vi "Set Scan Engine Active.vi"(8 "error in (no error)":errorcluster) -> (0 "error out":errorcluster)   [LabVIEW 2016]
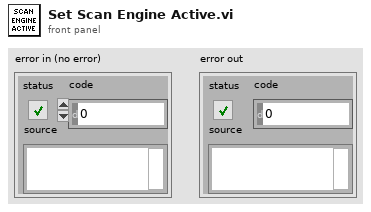
[diagram p1: front panel]
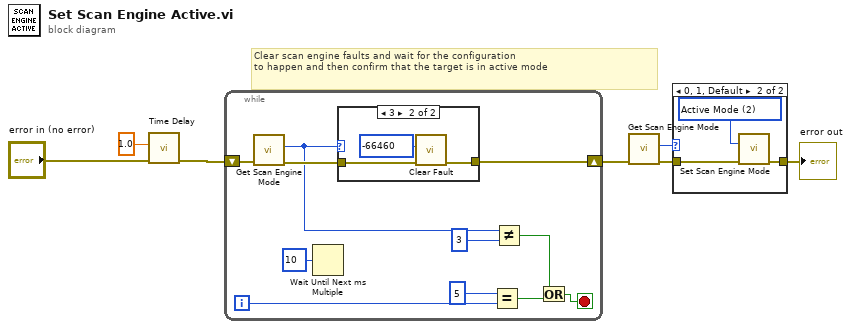
[diagram p0: block diagram]
diagram:
  # "Clear scan engine faults and wait for the configuration\nto happen and then confirm that the target is in active mode"
  n1 = call "Time Delay"("error in (no error)"="error in (no error)", "Delay Time (s)"=1.0) -> ("error out"=w5:errorcluster)  [unwired: 9 in]
  n2 = while {
    shift-right: [w8] -> w3
    shift-left: w5 -> [w18]
    i -> [w13]
    stop <- w16 stop-if-true
    n3 = call <vilib>:"Get Scan Engine Mode.vi"("error in (no error)"=w18) -> ("error out"=w17:errorcluster, "mode"=w9:i32)  [unwired: 9 in]
    n4 = Wait Until Next ms Multiple(millisecond multiple=u32 10) -> ()  [unwired: 1 out]
    n5 = case shown="3" w9 {
      tunnel: w17 -> [w19 w20]
      tunnel: [w19 w22] -> w8
      frame 0, Default {
      }
      frame 3 {
        n6 = call <vilib>:"Clear Fault.vi"("error in (no error)"=w20, "fault code"=-66460) -> ("error out"=w22:errorcluster)  [unwired: 9 in]
      }
    }
    n7 = Equal?(x=5, y=w13) -> (x = y?=w11:bool)
    n8 = Not Equal?(x=w9, y=3) -> (x != y?=w15:bool)
    n9 = Or(x=w15, y=w11) -> (x .or. y?=w16:bool)
  }
  n10 = call <vilib>:"Get Scan Engine Mode.vi"("error in (no error)"=w3) -> ("error out"=w2:errorcluster, "mode"=w1:i32)  [unwired: 9 in]
  n11 = case shown="0, 1, Default" w1 {
    tunnel: w2 -> [w23 w25]
    tunnel: [w23 w24] -> w7
    frame 2 {
    }
    frame 0, 1, Default {
      w26 = 2 items=["Configuration Mode"=1, "Active Mode"=2] ("mode (Active Mode)")
      n12 = call <vilib>:"Set Scan Engine Mode.vi"("mode (Active Mode)"=w26, "error in (no error)"=w25) -> ("error out"=w24:errorcluster)  [unwired: 13 in]
    }
  }
  "error out" <- w7
